vi "OPEN.vi"(8 "error in (no error)":errorcluster, 11 "VISA resource name":refnum<visa-resource-name>) -> (0 "error out":errorcluster, 1 "B":dbl, 2 "G":dbl, 3 "VISA resource name out":refnum<visa-resource-name>)   [LabVIEW 2016]
panel:
  in  "Enable Short Correction (F: Disable)":bool
  in  "Short Supplementary Threshold (0)":dbl
  in  "Short Capacitance Threshold (0)":dbl
  in  "Short Correction Type (0: Resistance- Reactance)":u16(ring) items=[" Resistance- Reactance", "Series Inductance- Series Resistance"]
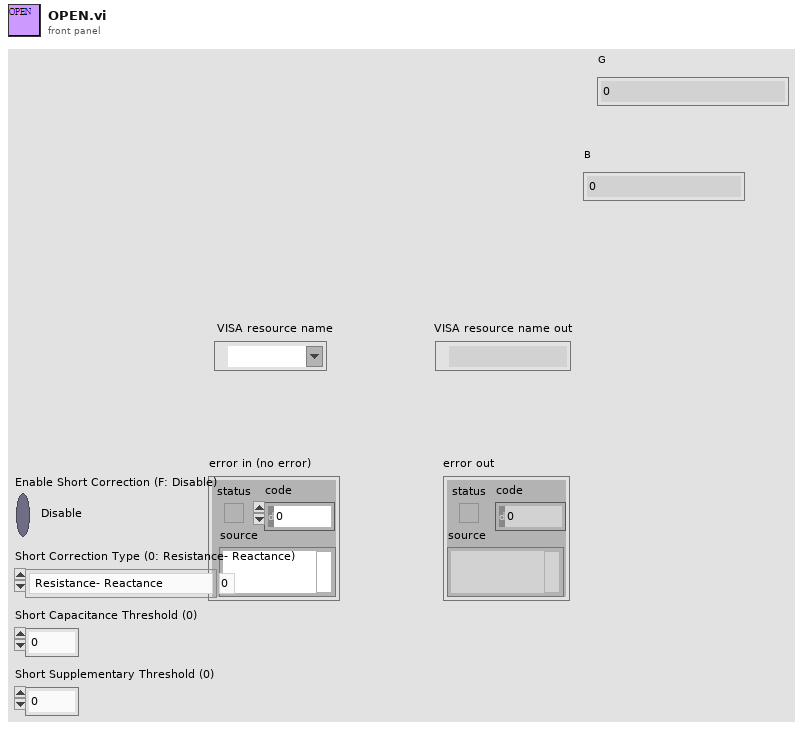
[diagram p1: front panel]
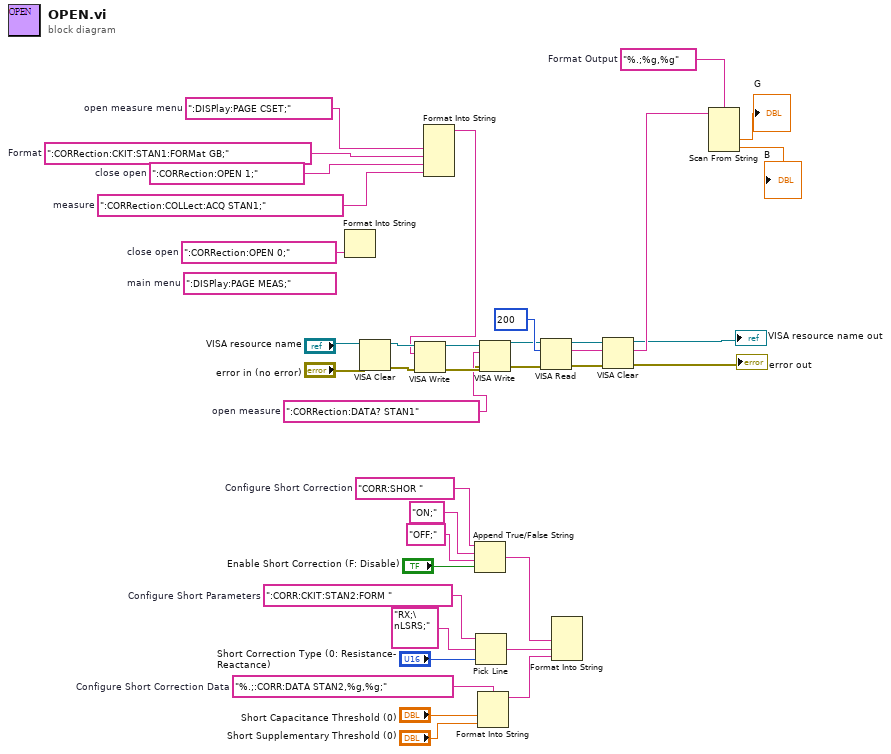
[diagram p0: block diagram]
diagram:
  w1 = ":CORRection:OPEN 1;"  # close open
  w9 = "%.;%g,%g"  # Format Output
  w16 = ":CORRection:DATA? STAN1"  # open measure
  w23 = ":CORRection:OPEN 0;"  # close open
  w24 = ":CORRection:COLLect:ACQ STAN1;"  # measure
  w2 = ":CORRection:CKIT:STAN1:FORMat GB;"  # Format
  (unwired) ":DISPlay:PAGE MEAS;"  # main menu
  w3 = ":DISPlay:PAGE CSET;"  # open measure menu
  w29 = "%.;:CORR:DATA STAN2,%g,%g;"  # Configure Short Correction Data
  w33 = ":CORR:CKIT:STAN2:FORM "  # Configure Short Parameters
  w37 = "CORR:SHOR "  # Configure Short Correction
  n1 = Format Into String(w23) -> ()  [unwired: 3 in, 2 out]
  n2 = VISA Clear(VISA resource name="VISA resource name", error in (no error)="error in (no error)") -> (VISA resource name out=w22:refnum<visa-resource-name>, error out=w21:errorcluster)
  n3 = Format Into String(w3, w2, w1, w24) -> (resulting string=w12:string)  [unwired: 3 in, 1 out]
  n4 = VISA Write(VISA resource name=w22, write buffer=w12, error in (no error)=w21) -> (VISA resource name out=w18:refnum<visa-resource-name>, error out=w17:errorcluster)  [unwired: 1 out]
  n5 = Append True/False String(1:"Enable Short Correction (F: Disable)", 2:"OFF;" ("true string"), 3:"ON;" ("true string"), 4:w37) -> (0:w26:string)
  n6 = Pick Line(string ("")=w33, multi-line string="RX;\nLSRS;", line index="Short Correction Type (0: Resistance- Reactance)") -> (output string=w27:string)
  n7 = Format Into String(format string=w29, "Short Capacitance Threshold (0)", "Short Supplementary Threshold (0)") -> (resulting string=w25:string)  [unwired: 2 in, 1 out]
  n8 = VISA Write(VISA resource name=w18, write buffer=w16, error in (no error)=w17) -> (VISA resource name out=w13:refnum<visa-resource-name>, error out=w14:errorcluster)  [unwired: 1 out]
  n9 = VISA Read(VISA resource name=w13, byte count=u32 200, error in (no error)=w14) -> (VISA resource name out=w7:refnum<visa-resource-name>, read buffer=w8:string, error out=w6:errorcluster)  [unwired: 1 out]
  n10 = Format Into String(w26, w27, w25) -> ()  [unwired: 3 in, 2 out]
  n11 = VISA Clear(VISA resource name=w7, error in (no error)=w6) -> (VISA resource name out=→"VISA resource name out":refnum<visa-resource-name>, error out=→"error out":errorcluster)
  n12 = Scan From String(format string=w9, input string=w8) -> (output 1=→"G":dbl, output 2=→"B":dbl)  [unwired: 4 in, 3 out]
